vi "runTestScenario.vi"(8 "error in (no error)":errorcluster, 11 "3.3VASupplyTest in":refnum<class "+3.3VASupplyTest.lvclass">) -> (0 "error out":errorcluster, 2 "TestExecution":T1, 3 "3.3VASupplyTest out":refnum<class "+3.3VASupplyTest.lvclass">)   [LabVIEW 2015, in "+3.3VASupplyTest.lvclass"]
uses:
  +3.3VASupplyTest.lvclass
  Typedefs/TestExecution.ctl
  Typedefs/WriteDataFileInput.ctl
  Typedefs/TestScenarioTypes.ctl
  Typedefs/WriteLogMessageInput.ctl
  Typedefs/PassFailTest.ctl
  +3.3VASupplyTest.lvclass/+3.3VASupplyTest.ctl
  Model/TestLog/ITestLog/ITestLog.lvclass
  Typedefs/ILCBTTypedefs.lvlib
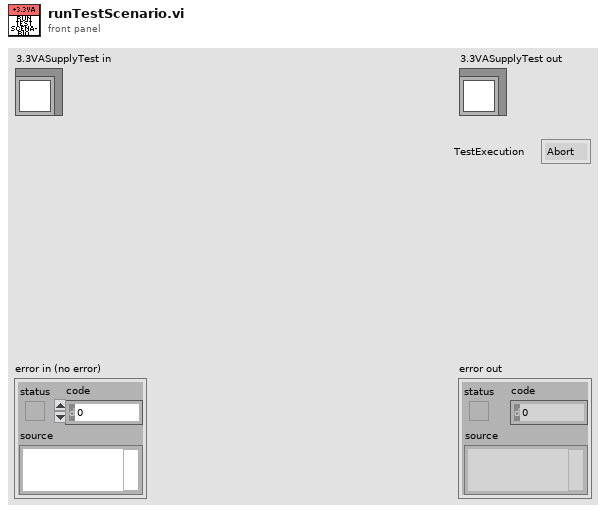
[diagram p1: front panel]
types:
  T1 = typedef "ILCBTTypedefs.lvlib/TestExecution.ctl" = enum16{"Abort", "Continue"}
  T2 = typedef "ILCBTTypedefs.lvlib/PassFailTest.ctl" = enum16{"Fail", "Pass", "NA"}
  T3 = typedef "ILCBTTypedefs.lvlib/WriteLogMessageInput.ctl" = cluster{"Test Scenario":T4, "Description":string, "Actual Value":string, "Data File":string, "Result":T2}
  T4 = typedef "ILCBTTypedefs.lvlib/TestScenarioTypes.ctl" = enum16{"+3.3VA Supply Test", "+3.3VD Supply Test", "+5VA Supply Test", "+5VD Supply Test"}
  T5 = typedef "ILCBTTypedefs.lvlib/WriteDataFileInput.ctl" = cluster{"Test Scenario":T4, "File Name":string, "Output":dbl[]}
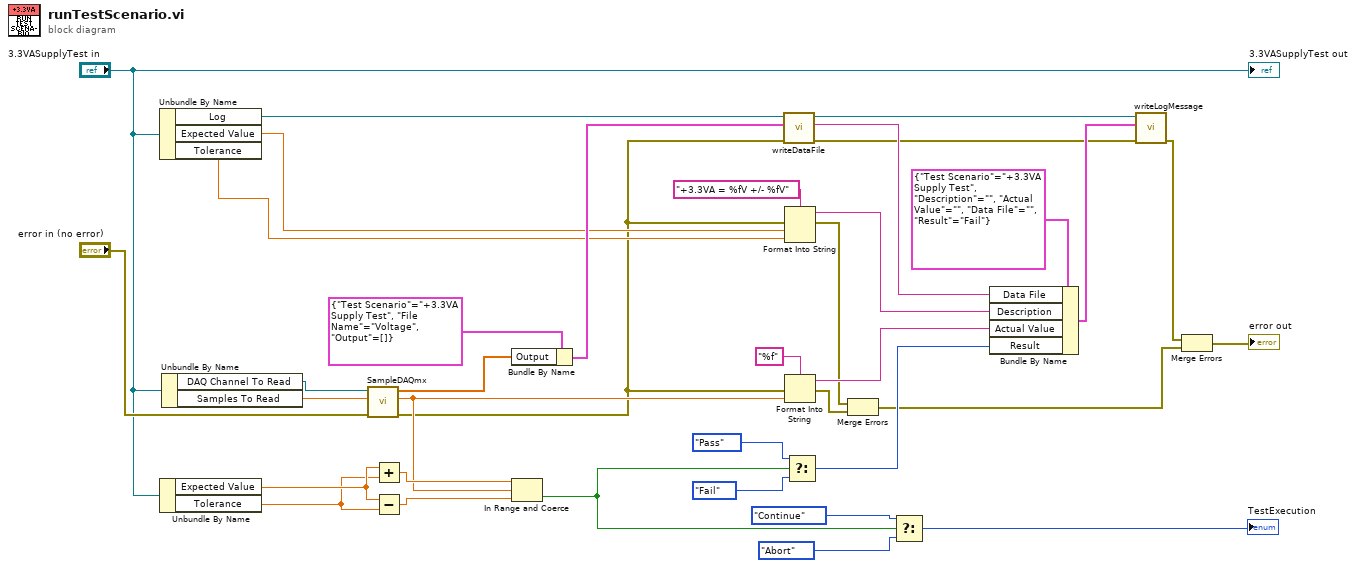
[diagram p0: block diagram]
diagram:
  n1 = Unbundle By Name("3.3VASupplyTest in") -> ("Log"=w36:refnum<class "ITestLog.lvclass">, "Expected Value"=w12:dbl[unit], "Tolerance"=w11:dbl[unit])
  n2 = Unbundle By Name("3.3VASupplyTest in") -> ("Expected Value"=w23:dbl[unit], "Tolerance"=w22:dbl[unit])
  n3 = Unbundle By Name("3.3VASupplyTest in") -> ("DAQ Channel To Read"=w27:refnum<k21>, "Samples To Read"=w26:dbl)
  n4 = call "SampleDAQmx.vi"("error in (no error)"="error in (no error)", "Samples To Read"=w26, "DAQ Channel To Read"=w27) -> ("error out"=w10:errorcluster, "Average"=w13:dbl, "Samples"=w35:dbl[])  [unwired: 6 in]
  n5 = Add(x=w23, y=w22) -> (x+y=w21:dbl[unit])
  n6 = Subtract(x=w23, y=w22) -> (x-y=w20:dbl[unit])
  n7 = Bundle By Name(cluster=T5 {"Test Scenario"=enum."+3.3VA Supply Test", "File Name"="Voltage", "Output"=[]} ("WriteDataFileInput"), "Output"=w35) -> (w24:T5)
  n8 = In Range and Coerce(upper limit=w21, x=w13, lower limit=w20) -> (In Range?=w15:bool)  [unwired: 1 out]
  n9 = call-dynamic "writeDataFile.vi"("error in (no error)"=w10, "WriteDataFileInput"=w24, "ITestLog in"=w36) -> ("error out"=w6:errorcluster, "Relative Path"=w9:string, "ITestLog out"=w30:refnum<class "ITestLog.lvclass">)  [unwired: 6 in]
  n10 = Format Into String(format string="+3.3VA = %fV +/- %fV", error in=w10, w12, w11) -> (resulting string=w8:string, error out=w5:errorcluster)  [unwired: 1 in]
  n11 = Format Into String(format string="%f", error in=w10, w13) -> (resulting string=w7:string, error out=w4:errorcluster)  [unwired: 1 in]
  n12 = Select(t=PassFailTest."Pass" ("Result"), s=w15, f=PassFailTest."Fail" ("Result")) -> (s? t:f=w31:T2)
  n13 = Merge Errors(w5, w4) -> (w1:errorcluster)
  n14 = Select(t=TestExecution."Continue" ("TestExecution"), s=w15, f=TestExecution."Abort" ("TestExecution")) -> (s? t:f=→"TestExecution":T1)
  n15 = Bundle By Name(cluster=T3 {"Test Scenario"=enum."+3.3VA Supply Test", "Description"="", "Actual Value"="", "Data File"="", "Result"=enum."Fail"} ("WriteLogMessageInput"), "Data File"=w9, "Description"=w8, "Actual Value"=w7, "Result"=w31) -> (w29:T3)
  n16 = call-dynamic "writeLogMessage.vi"("error in (no error)"=w6, "WriteLogMessageInput"=w29, "ITestLog in"=w30) -> ("error out"=w2:errorcluster)  [unwired: 7 in, 1 out]
  n17 = Merge Errors(w2, w1) -> (→"error out":errorcluster)
  "3.3VASupplyTest out" <- "3.3VASupplyTest in"
